vi "Fixed Counter with Semaphore.vi"() -> ()   [LabVIEW 2012]
panel:
  out "Running Total":i32
  in  "Stop Button":bool
  out "Loop Count Difference":i32
  out "Loop Count 2":i32
  out "Loop Count 1":i32
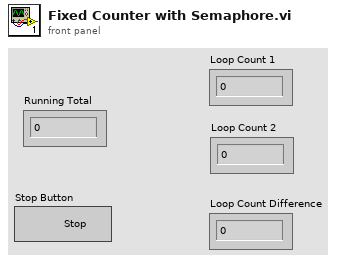
[diagram p1: front panel]
types:
  T1 = typedef "Semaphore RefNum" = refnum<k1>
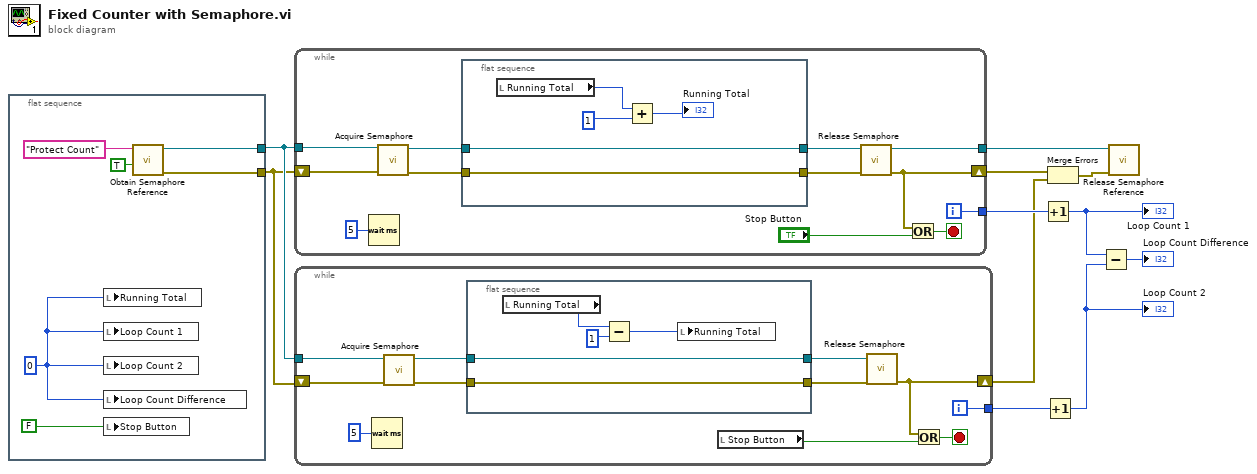
[diagram p0: block diagram]
diagram:
  n1 = flat-sequence {
    tunnel: [w15] -> w5
    tunnel: [w14] -> w6
    frame #0 {
      w12 = 0 ("Running Total")
      n2 = local write "Running Total"(w12) -> ()
      n3 = local write "Loop Count 1"(w12) -> ()
      n4 = local write "Loop Count 2"(w12) -> ()
      n5 = local write "Loop Count Difference"(w12) -> ()
      n6 = local write "Stop Button"(FALSE ("Stop Button")) -> ()
      n7 = call <vilib>:"Obtain Semaphore Reference.vi"("create if not found (T)"=TRUE, "name (unnamed)"="Protect Count") -> ("error out"=w15:errorcluster, "semaphore"=w14:T1)  [unwired: 3 in, 1 out]
    }
  }
  n8 = while {
    tunnel: [w27] -> w11
    tunnel: w6 -> [w26]
    tunnel: [w20] -> w4
    shift-right: [w18] -> w3
    shift-left: w5 -> [w25]
    i -> [w27]
    stop <- w19 stop-if-true
    n9 = Wait (ms)(milliseconds to wait=u32 5) -> ()  [unwired: 1 out]
    n10 = call <vilib>:"Acquire Semaphore.vi"("error in (no error)"=w25, "semaphore"=w26) -> ("error out"=w24:errorcluster, "semaphore out"=w22:T1)  [unwired: 3 in, 1 out]
    n11 = flat-sequence {
      tunnel: w24 -> [w32]
      tunnel: [w32] -> w23
      tunnel: w22 -> [w31]
      tunnel: [w31] -> w21
      frame #0 {
        n12 = local read "Running Total"() -> (w30:i32)
        n13 = Add(x=w30, y=1 ("x")) -> (x+y=→"Running Total":i32)
      }
    }
    n14 = call <vilib>:"Release Semaphore.vi"("error in (no error)"=w23, "semaphore"=w21) -> ("error out"=w18:errorcluster, "semaphore out"=w20:T1)  [unwired: 4 in]
    n15 = Or(x=w18, y="Stop Button") -> (x .or. y?=w19:bool)
  }
  n16 = while {
    tunnel: [w44] -> w10
    tunnel: w6 -> [w43]
    shift-right: [w35] -> w1
    shift-left: w5 -> [w42]
    i -> [w44]
    stop <- w38 stop-if-true
    n17 = Wait (ms)(milliseconds to wait=u32 5) -> ()  [unwired: 1 out]
    n18 = call <vilib>:"Acquire Semaphore.vi"("error in (no error)"=w42, "semaphore"=w43) -> ("error out"=w41:errorcluster, "semaphore out"=w40:T1)  [unwired: 3 in, 1 out]
    n19 = flat-sequence {
      tunnel: w41 -> [w46]
      tunnel: w40 -> [w47]
      tunnel: [w47] -> w39
      tunnel: [w46] -> w36
      frame #0 {
        n20 = local read "Running Total"() -> (w50:i32)
        n21 = Subtract(x=w50, y=1 ("x")) -> (x-y=w48:i32)
        n22 = local write "Running Total"(w48) -> ()
      }
    }
    n23 = local read "Stop Button"() -> (w37:bool)
    n24 = call <vilib>:"Release Semaphore.vi"("error in (no error)"=w36, "semaphore"=w39) -> ("error out"=w35:errorcluster)  [unwired: 4 in, 1 out]
    n25 = Or(x=w35, y=w37) -> (x .or. y?=w38:bool)
  }
  n26 = Increment(x=w11) -> (x+1=w9:i32)
  "Loop Count 1" <- w9
  n27 = Increment(x=w10) -> (x+1=w8:i32)
  "Loop Count 2" <- w8
  n28 = Merge Errors(w3, w1) -> (w2:errorcluster)
  n29 = Subtract(x=w9, y=w8) -> (x-y=→"Loop Count Difference":i32)
  n30 = call <vilib>:"Release Semaphore Reference.vi"("error in (no error)"=w2, "semaphore"=w4) -> ()  [unwired: 8 in, 2 out]
